vi "Compile Protocol.vi"(8 "error in (no error)":errorcluster, 10 "Protocol":refnum<class "Protocol.lvclass">, 11 "AutomationContext in":refnum<class "AutomationContext.lvclass">) -> (0 "error out":errorcluster, 3 "AutomationContext out":refnum<class "AutomationContext.lvclass">)   [LabVIEW 2023, in "Automation.lvlib" / "AutomationContext.lvclass"]
uses:
  AutomationContext.lvclass
  Protocol/Protocol.lvclass
  Intent Action.ctl
  Resources/Type Defs/Camera Settings.ctl
  AutomationContext.lvclass/AutomationContext.ctl
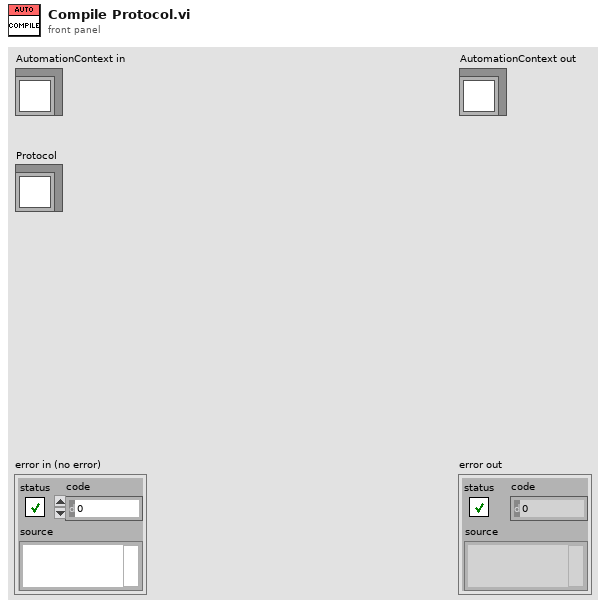
[diagram p1: front panel]
types:
  T1 = typedef "Camera Settings.ctl" = cluster{"Exposure Time (ms)":dbl, "Binning":enum16{"1x1", "2x2", "4x4"}, "Scan Mode":i32, "Frames to Acquire":dbl, "Pixel Correction":bool, "Frames to Skip":u32, "File Path":path, "Duty cycle":dbl, "ALEX":bool, "Shutter Enable":bool[], "fluidics trigger, ms (0=disabled)":dbl, "Bit Depth":u16, "Image Width (px)":u16, "Image Height (px)":u16, "Horizontal Offset (px)":u16, "Vertical Offset (px)":u16}
  T2 = cluster{"Camera Settings":T1, "Injection Countdown":bool}
  T3 = typedef "Automation.lvlib/AutomationContext.lvclass/Intent Action.ctl" = enum16{"Next Field", "Next Lane", "Set Power", "Reset Power", "Autofocus", "Start Streaming", "Delay", "Finish Run", "Open Shutter", "Close Shutter"}
  T4 = typedef "Movie Series.ctl" = cluster{"Fields":i32, "Lanes":i32, "Acquisition type":T5, "Sweep":T6}
  T5 = typedef "Movie auto-numbering.ctl" = enum16{"Single movie", "Movie series", "Multi-lane series", "Sweep Parameter"}
  T6 = typedef "Param Sweep.ctl" = cluster{"Parameter":enum16{"Laser Power (mW)", "Exposure Time (ms)"}, "Values":u32[], "Repeats":u32}
  T7 = typedef "Movie Settings.ctl" = cluster{"Camera Settings":T1, "Auto-Advance":bool, "Auto Focus":bool, "Injection Countdown":bool, "Particle Count Threshold":i32, "Laser Power (mW)":u32}
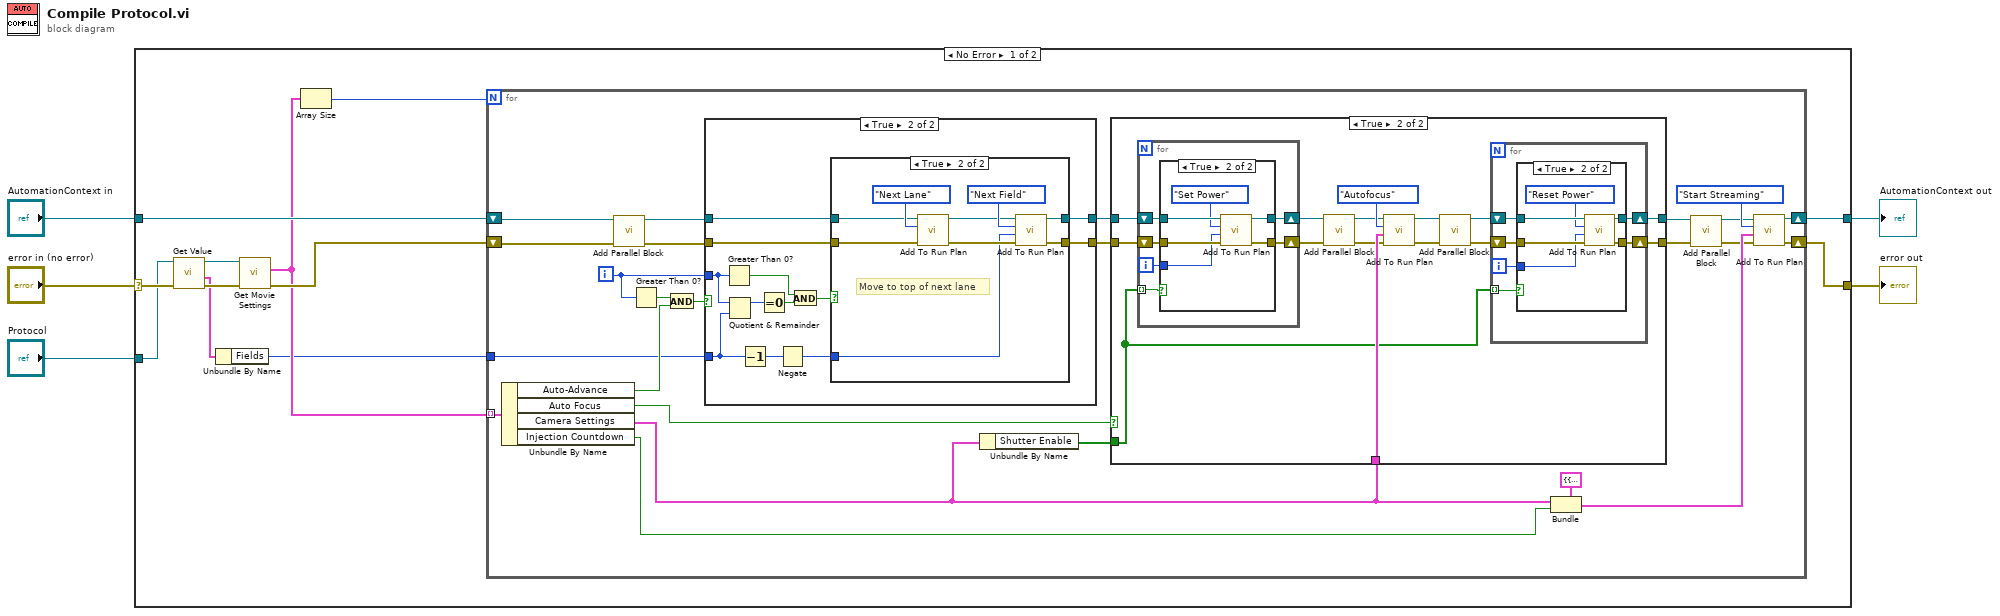
[diagram p0: block diagram]
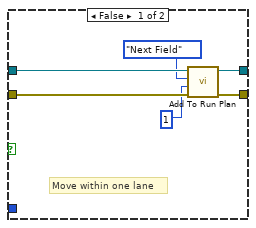
[diagram p3: hidden frame]
diagram:
  n1 = case shown="No Error" "error in (no error)" {
    selector: "error in (no error)" -> [w11 w118]
    tunnel: [w15 w118] -> w4
    tunnel: [w16 w117] -> w2
    tunnel: "AutomationContext in" -> [w17 w117]
    tunnel: "Protocol" -> [w8 _]
    frame No Error {
      n2 = call "Get Value.vi"("error in (no error)"=w11, "Protocol in"=w8) -> ("error out"=w10:errorcluster, "Movie Series"=w6:T4, "Protocol out"=w9:refnum<class "Protocol.lvclass">)  [unwired: 6 in, 1 out]
      n3 = Unbundle By Name(w6) -> ("Fields"=w7:i32)
      n4 = call "Get Movie Settings.vi"("error in (no error)"=w10, "Protocol in"=w9) -> ("error out"=w14:errorcluster, "Movie Settings Array"=w12:T7[])  [unwired: 7 in, 1 out]
      n5 = Array Size(array=w12) -> (size(s)=w13:i32)
      n6 = for {
        N: w13 -> [_]
        shift-right: [w41] -> w16
        shift-left: w17 -> [w27]
        shift-right: [w42] -> w15
        shift-left: w14 -> [w26]
        tunnel: w12 -> [w23] mode=indexing
        tunnel: w7 -> [w20]
        i -> [w34]
        n7 = Unbundle By Name(w23) -> ("Auto-Advance"=w22:bool, "Auto Focus"=w18:bool, "Camera Settings"=w19:T1, "Injection Countdown"=w21:bool)
        n8 = call "Add Parallel Block.vi"("error in (no error)"=w26, "AutomationContext in"=w27) -> ("error out"=w25:errorcluster, "AutomationContext out"=w24:refnum<class "AutomationContext.lvclass">)  [unwired: 8 in]
        n9 = Greater Than 0?(x=w34) -> (x > 0?=w39:bool)
        n10 = And(x=w39, y=w22) -> (x .and. y?=w40:bool)
        n11 = case shown="True" w40 {
          tunnel: w34 -> [_ w55]
          tunnel: w20 -> [_ w49]
          tunnel: w24 -> [w44 w46]
          tunnel: [w44 w48] -> w38
          tunnel: [w43 w47] -> w37
          tunnel: w25 -> [w43 w45]
          frame False {
            # "Stage disabled or first movie"
          }
          frame True {
            n12 = Greater Than 0?(x=w55) -> (x > 0?=w54:bool)
            n13 = Quotient & Remainder(x=w55, y=w49) -> (x-y*floor(x/y)=w52:i32)  [unwired: 1 out]
            n14 = Decrement(x=w49) -> (x-1=w50:i32)
            n15 = Equal To 0?(x=w52) -> (x = 0?=w53:bool)
            n16 = Negate(x=w50) -> (-x=w51:i32)
            n17 = And(x=w54, y=w53) -> (x .and. y?=w56:bool)
            n18 = case shown="True" w56 {
              tunnel: w51 -> [_ w64]
              tunnel: w46 -> [w59 w63]
              tunnel: [w60 w69] -> w48
              tunnel: w45 -> [w62 w68]
              tunnel: [w61 w70] -> w47
              frame False {
                # "Move within one lane"
                n19 = call "Add To Run Plan.vi"("error in (no error)"=w62, "Parameters"=1, "Action"=Intent_Action."Next Field", "AutomationContext in"=w59) -> ("error out"=w61:errorcluster, "AutomationContext out"=w60:refnum<class "AutomationContext.lvclass">)  [unwired: 6 in]
              }
              frame True {
                # "Move to top of next lane"
                n20 = call "Add To Run Plan.vi"("error in (no error)"=w68, "Action"=Intent_Action."Next Lane", "AutomationContext in"=w63) -> ("error out"=w67:errorcluster, "AutomationContext out"=w66:refnum<class "AutomationContext.lvclass">)  [unwired: 7 in]
                n21 = call "Add To Run Plan.vi"("error in (no error)"=w67, "Parameters"=w64, "Action"=Intent_Action."Next Field", "AutomationContext in"=w66) -> ("error out"=w70:errorcluster, "AutomationContext out"=w69:refnum<class "AutomationContext.lvclass">)  [unwired: 6 in]
              }
            }
          }
        }
        n22 = Unbundle By Name(w19) -> ("Shutter Enable"=w33:bool[])
        n23 = case shown="True" w18 {
          tunnel: w38 -> [w73 w85]
          tunnel: [w73 w86] -> w30
          tunnel: w37 -> [w72 w88]
          tunnel: [w72 w87] -> w31
          tunnel: w19 -> [_ w83]
          tunnel: w33 -> [_ w82]
          frame False {
            # "Autofocus disabled"
          }
          frame True {
            n24 = for {
              shift-right: [w107] -> w80
              shift-left: w88 -> [w108]
              shift-right: [w106] -> w81
              shift-left: w85 -> [w105]
              tunnel: w82 -> [w104] mode=indexing
              i -> [w103]
              n25 = case shown="True" w104 {
                tunnel: w108 -> [w109 w116]
                tunnel: [w109 w115] -> w107
                tunnel: [w110 w114] -> w106
                tunnel: w105 -> [w110 w113]
                tunnel: w103 -> [_ w111]
                frame False {
                }
                frame True {
                  n26 = call "Add To Run Plan.vi"("error in (no error)"=w116, "Parameters"=w111, "Action"=Intent_Action."Set Power", "AutomationContext in"=w113) -> ("error out"=w115:errorcluster, "AutomationContext out"=w114:refnum<class "AutomationContext.lvclass">)  [unwired: 6 in]
                }
              }
            }
            n27 = call "Add Parallel Block.vi"("error in (no error)"=w80, "AutomationContext in"=w81) -> ("error out"=w79:errorcluster, "AutomationContext out"=w78:refnum<class "AutomationContext.lvclass">)  [unwired: 8 in]
            n28 = call "Add To Run Plan.vi"("error in (no error)"=w79, "Parameters"=w83, "Action"=Intent_Action."Autofocus", "AutomationContext in"=w78) -> ("error out"=w77:errorcluster, "AutomationContext out"=w76:refnum<class "AutomationContext.lvclass">)  [unwired: 6 in]
            n29 = call "Add Parallel Block.vi"("error in (no error)"=w77, "AutomationContext in"=w76) -> ("error out"=w74:errorcluster, "AutomationContext out"=w75:refnum<class "AutomationContext.lvclass">)  [unwired: 8 in]
            n30 = for {
              shift-right: [w93] -> w87
              shift-left: w74 -> [w94]
              shift-right: [w92] -> w86
              shift-left: w75 -> [w91]
              tunnel: w82 -> [w89] mode=indexing
              i -> [w90]
              n31 = case shown="True" w89 {
                tunnel: w94 -> [w95 w102]
                tunnel: [w95 w101] -> w93
                tunnel: [w96 w100] -> w92
                tunnel: w91 -> [w96 w99]
                tunnel: w90 -> [_ w97]
                frame False {
                }
                frame True {
                  n32 = call "Add To Run Plan.vi"("error in (no error)"=w102, "Parameters"=w97, "Action"=Intent_Action."Reset Power", "AutomationContext in"=w99) -> ("error out"=w101:errorcluster, "AutomationContext out"=w100:refnum<class "AutomationContext.lvclass">)  [unwired: 6 in]
                }
              }
            }
          }
        }
        n33 = Bundle(cluster=T2 {"Camera Settings"={"Exposure Time (ms)"=0.0, "Binning"=enum."1x1", "Scan Mode"=0, "Frames to Acquire"=0.0, "Pixel Correction"=FALSE, "Frames to Skip"=0, "File Path"=path "", "Duty cycle"=0.0, "ALEX"=FALSE, "Shutter Enable"=[], "fluidics trigger, ms (0=disabled)"=0.0, "Bit Depth"=0, "Image Width (px)"=0, "Image Height (px)"=0, "Horizontal Offset (px)"=0, "Vertical Offset (px)"=0}, "Injection Countdown"=FALSE}, "Camera Settings"=w19, "Injection Countdown"=w21) -> (w32:T2)
        n34 = call "Add Parallel Block.vi"("error in (no error)"=w31, "AutomationContext in"=w30) -> ("error out"=w28:errorcluster, "AutomationContext out"=w29:refnum<class "AutomationContext.lvclass">)  [unwired: 8 in]
        n35 = call "Add To Run Plan.vi"("error in (no error)"=w28, "Parameters"=w32, "Action"=Intent_Action."Start Streaming", "AutomationContext in"=w29) -> ("error out"=w42:errorcluster, "AutomationContext out"=w41:refnum<class "AutomationContext.lvclass">)  [unwired: 6 in]
      }
    }
    frame Error {
    }
  }
  "error out" <- w4
  "AutomationContext out" <- w2
